vi "NetComm_CAN_Send.vi"(6 "Period (ms)":i32, 8 "error in (no error)":errorcluster, 9 "Data":u8[](array[numeric]), 10 "Message ID":u32 format="%.0x") -> (0 "error out":errorcluster)   [LabVIEW 2017]
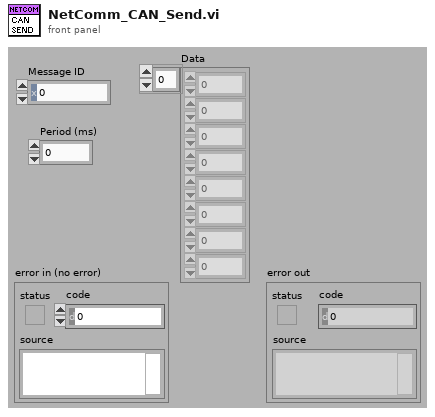
[diagram p1: front panel]
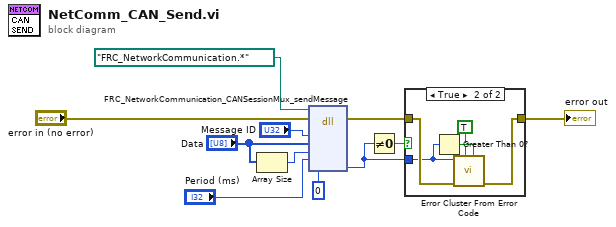
[diagram p0: block diagram]
diagram:
  n1 = Array Size(array="Data") -> (size(s)=w4:i32)
  n2 = dll-call lib="FRC_NetworkCommunication.*" fn="FRC_NetworkCommunication_CANSessionMux_sendMessage"(path in=path "FRC_NetworkCommunication.*", error in="error in (no error)", "messageID"="Message ID", "data"="Data", "dataSize"=w4, "periodMs"="Period (ms)", "status"=0) -> (error out=w7:errorcluster, "status"=w6:i32)  [unwired: 6 in, 1 out]
  n3 = Not Equal To 0?(x=w6) -> (x != 0?=w10:bool)
  n4 = case shown="True" w10 {
    tunnel: w7 -> [w12 w17]
    tunnel: w6 -> [_ w15]
    tunnel: [w12 w14] -> w11
    frame False {
    }
    frame True {
      n5 = Greater Than 0?(x=w15) -> (x > 0?=w16:bool)
      n6 = call <vilib>:"Error Cluster From Error Code.vi"("is warning? (False)"=w16, "show call chain? (False)"=TRUE, "error in (no error)"=w17, "error code (0)"=w15) -> ("error out"=w14:errorcluster)  [unwired: 5 out]
    }
  }
  "error out" <- w11
